vi "WindSimulator.vi"(0 "Sine Mean (m/s)":dbl, 1 "Sine Amp (m/s)":dbl, 2 "Sine Freq (Hz)":dbl, 3 "Ramp Start u(m/s)":dbl, 4 "Ramp End u(m/s)":dbl, 5 "Ramp Time (s)":dbl, 6 "Const. Amp (m/s)":dbl, 7 "Wind Simulation":T1, 9 "Loop Time (s)":dbl) -> (14 "Wind Speed (m/s)":dbl, 19 "Ramp time (s)":dbl)   [LabVIEW 2018]
uses:
  Clusters/WindSimCtrl.ctl
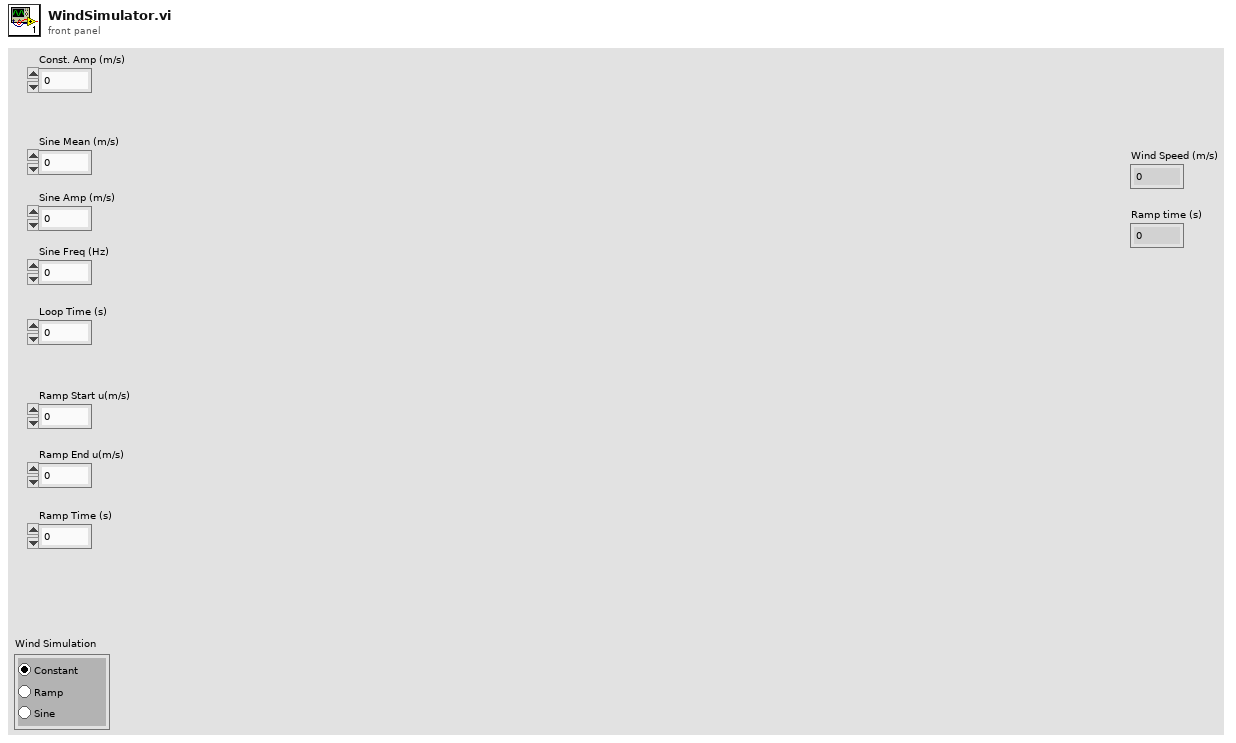
[diagram p1: front panel]
types:
  T1 = typedef "WindSimCtrl.ctl" = enum32{"Constant", "Ramp", "Sine"}
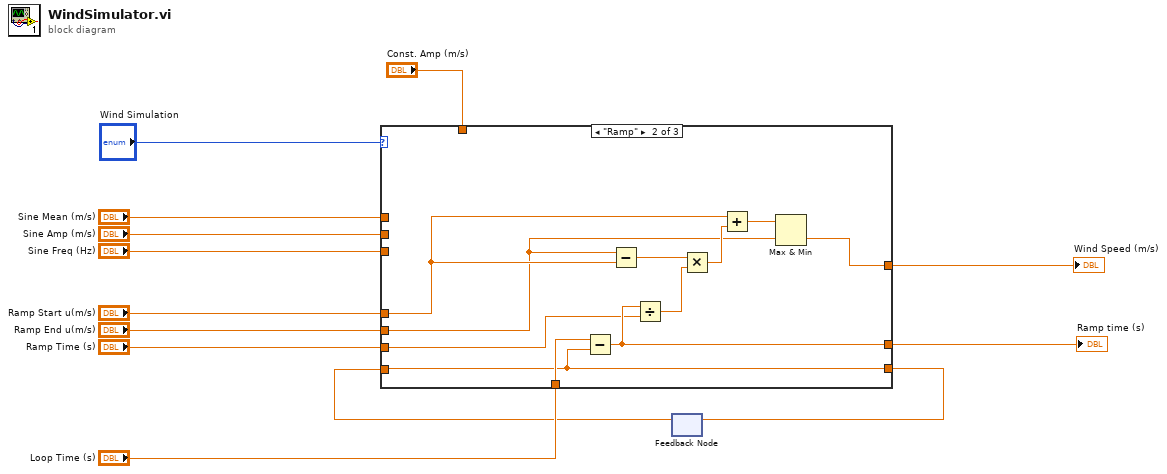
[diagram p0: block diagram]
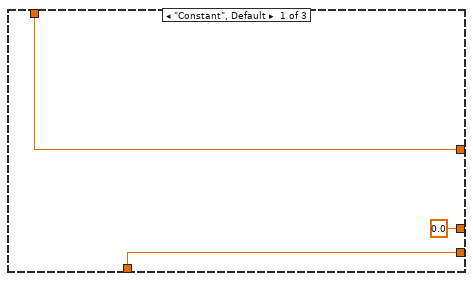
[diagram p2: hidden frame]
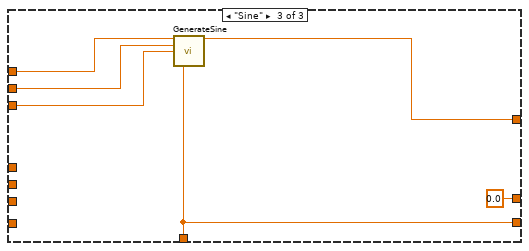
[diagram p3: hidden frame]
diagram:
  n1 = feedback #1() -> (w2:dbl)  [unwired: 1 in]
  n2 = case shown="\"Ramp\"" "Wind Simulation" {
    tunnel: "Const. Amp (m/s)" -> [w16 _ _]
    tunnel: [w16 w17 w31] -> w11
    tunnel: "Sine Mean (m/s)" -> [_ _ w33]
    tunnel: "Sine Amp (m/s)" -> [_ _ w32]
    tunnel: "Sine Freq (Hz)" -> [_ _ w30]
    tunnel: "Loop Time (s)" -> [w15 w27 w29]
    tunnel: "Ramp Start u(m/s)" -> [_ w19 _]
    tunnel: "Ramp End u(m/s)" -> [_ w18 _]
    tunnel: "Ramp Time (s)" -> [_ w22 _]
    tunnel: [w15 w26 w29] -> w3
    tunnel: w2 -> [_ w26 _]
    tunnel: [0.0 w23 0.0] -> w1
    frame "Constant", Default {
    }
    frame "Ramp" {
      n3 = Subtract(x=w27, y=w26) -> (x-y=w23:dbl)
      n4 = Subtract(x=w18, y=w19) -> (x-y=w25:dbl)
      n5 = Divide(x=w23, y=w22) -> (x/y=w24:dbl)
      n6 = Multiply(x=w25, y=w24) -> (x*y=w21:dbl)
      n7 = Add(x=w19, y=w21) -> (x+y=w20:dbl)
      n8 = Max & Min(x=w20, y=w18) -> (min(x,y)=w17:dbl)  [unwired: 1 out]
    }
    frame "Sine" {
      n9 = call "GenerateSine.vi"("Mean"=w33, "Amplitude"=w32, "frequency (f)"=w30, "time (s)"=w29) -> ("sine out"=w31:dbl)  [unwired: 11 in]
    }
  }
  "Wind Speed (m/s)" <- w11
  "Ramp time (s)" <- w1
  n10 = feedback-in #1(w3) -> ()
